vi "Deney 3.1.vi"() -> ()   [LabVIEW 2018]
panel:
  out "Q1":bool
  in  "stop":bool
  out "Q2":bool
  out "6":bool
  out "5":bool
  out "4":bool
  out "3":bool
  out "1":bool
  out "2":bool
  out "Q0":bool
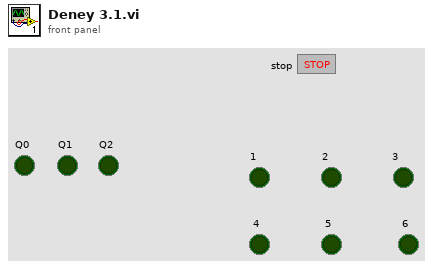
[diagram p1: front panel]
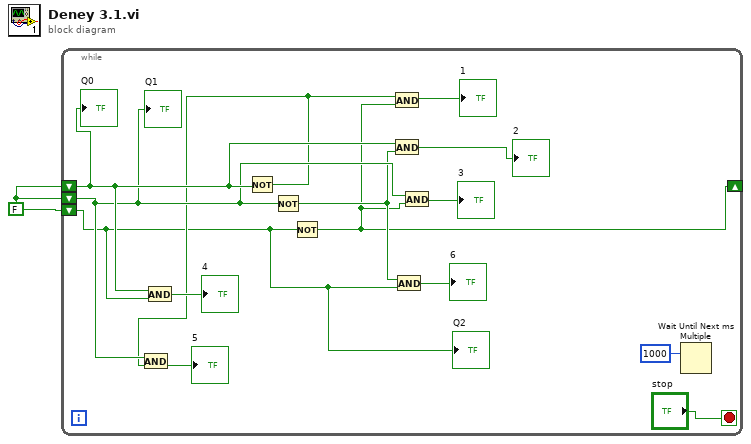
[diagram p0: block diagram]
diagram:
  w1 = FALSE
  n1 = while {
    shift-right: [w2] -> _
    shift-left: w1 -> [w10]
    shift-left: w1 -> [w9]
    shift-left: w1 -> [w3]
    stop <- "stop" stop-if-true
    n2 = And(x=w10, y=w3) -> (x .and. y?=→"4":bool)
    n3 = Not(x=w10) -> (.not. x?=w5:bool)
    n4 = And(x=w9, y=w5) -> (x .and. y?=→"5":bool)
    n5 = Not(x=w9) -> (.not. x?=w4:bool)
    n6 = Not(x=w3) -> (.not. x?=w2:bool)
    n7 = And(x=w5, y=w2) -> (x .and. y?=→"1":bool)
    n8 = And(x=w10, y=w4) -> (x .and. y?=→"2":bool)
    n9 = And(x=w4, y=w3) -> (x .and. y?=→"6":bool)
    n10 = And(x=w9, y=w2) -> (x .and. y?=→"3":bool)
    n11 = Wait Until Next ms Multiple(millisecond multiple=1000) -> ()  [unwired: 1 out]
    "Q0" <- w10
    "Q2" <- w3
    "Q1" <- w9
  }
